vi "Code Page Table.vi"() -> (3 "Code Page Table":T1(array[cluster])=[{"Name"="Thai", "Tag"="th", "Code Page"=874}, {"Name"="Japanese", "Tag"="ja", "Code Page"=932}, {"Name"="Chinese (Simp)", "Tag"="zh-cn", "Code Page"=936}, {"Name"="Korean", "Tag"="ko", "Code Page"=949}, {"Name"="Chinese (Trad)", "Tag"="zh-tw", "Code Page"=950}, {"Name"="Czech", "Tag"="cs", "Code Page"=1250}, {"Name"="Slovak", "Tag"="sk", "Code Page"=1250}, {"Name"="Polish", "Tag"="pl", "Code Page"=1250}, {"Name"="Hungarian", "Tag"="hu", "Code Page"=1250}, {"Name"="Slovene", "Tag"="sl", "Code Page"=1250}, {"Name"="Bosnian", "Tag"="bs", "Code Page"=1250}, {"Name"="Croatian", "Tag"="hr", "Code Page"=1250}, {"Name"="Serbian", "Tag"="sr", "Code Page"=1250}, {"Name"="Romanian", "Tag"="ro", "Code Page"=1250}, {"Name"="Albanian", "Tag"="sq", "Code Page"=1250}, {"Name"="Russian", "Tag"="ru", "Code Page"=1251}, {"Name"="Bulgarian", "Tag"="bg", "Code Page"=1251}, {"Name"="Macedonian", "Tag"="mk", "Code Page"=1251}, {"Name"="Ukrainian", "Tag"="uk", "Code Page"=1251}, {"Name"="Afrikaans", "Tag"="af", "Code Page"=1252}, {"Name"="Basque", "Tag"="eu", "Code Page"=1252}, {"Name"="Catalan", "Tag"="ca", "Code Page"=1252}, {"Name"="Danish", "Tag"="da", "Code Page"=1252}, {"Name"="Dutch", "Tag"="nl", "Code Page"=1252}, {"Name"="English", "Tag"="en", "Code Page"=1252}, {"Name"="Faroese", "Tag"="fo", "Code Page"=1252}, {"Name"="Finnish", "Tag"="fi", "Code Page"=1252}, {"Name"="French", "Tag"="fr", "Code Page"=1252}, {"Name"="Galician", "Tag"="gl", "Code Page"=1252}, {"Name"="German", "Tag"="ge", "Code Page"=1252}, {"Name"="Icelandic", "Tag"="is", "Code Page"=1252}, {"Name"="Irish", "Tag"="ga", "Code Page"=1252}, {"Name"="Italian", "Tag"="it", "Code Page"=1252}, {"Name"="Norwegian", "Tag"="no", "Code Page"=1252}, {"Name"="Portuguese", "Tag"="pt", "Code Page"=1252}, {"Name"="Scottish", "Tag"="gd", "Code Page"=1252}, {"Name"="Spanish", "Tag"="es", "Code Page"=1252}, {"Name"="Swedish", "Tag"="sv", "Code Page"=1252}, {"Name"="Greek", "Tag"="el", "Code Page"=1253}, {"Name"="Turkish", "Tag"="tr", "Code Page"=1254}, {"Name"="Hebrew", "Tag"="he", "Code Page"=1255}, {"Name"="Farsi", "Tag"="fa", "Code Page"=1256}, {"Name"="Latvian", "Tag"="lv", "Code Page"=1257}, {"Name"="Lithuanian", "Tag"="lt", "Code Page"=1257}, {"Name"="Estonian", "Tag"="et", "Code Page"=1257}, {"Name"="Vietnamese", "Tag"="vt", "Code Page"=1258}])   [LabVIEW 2013, in "SET Project Data.lvlib"]
uses:
  SET Project Data.lvlib
panel:
  # "List of all supported languages. This should be stored in a config file but this should\ndo for now."
  # "Sources:\n1) List of ISO 639-1 codes - Wikipedia, the free encyclopedia\nhttp://en.wikipedia.org/wiki/List_of_ISO_639-1_codes\n\n2) Israel Science and Technology Homepage - Windows Locale Codes - Sortable list\nhttp://www.science.co.il/Language/Locale-codes.asp"
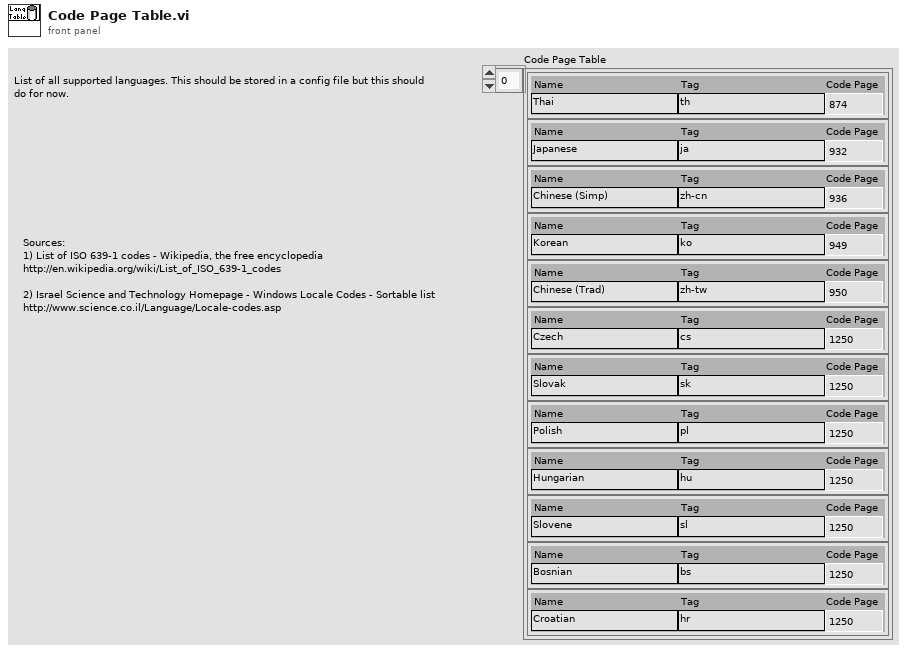
[diagram p1: front panel]
types:
  T1 = cluster{"Name":string, "Tag":string, "Code Page":u16}[]
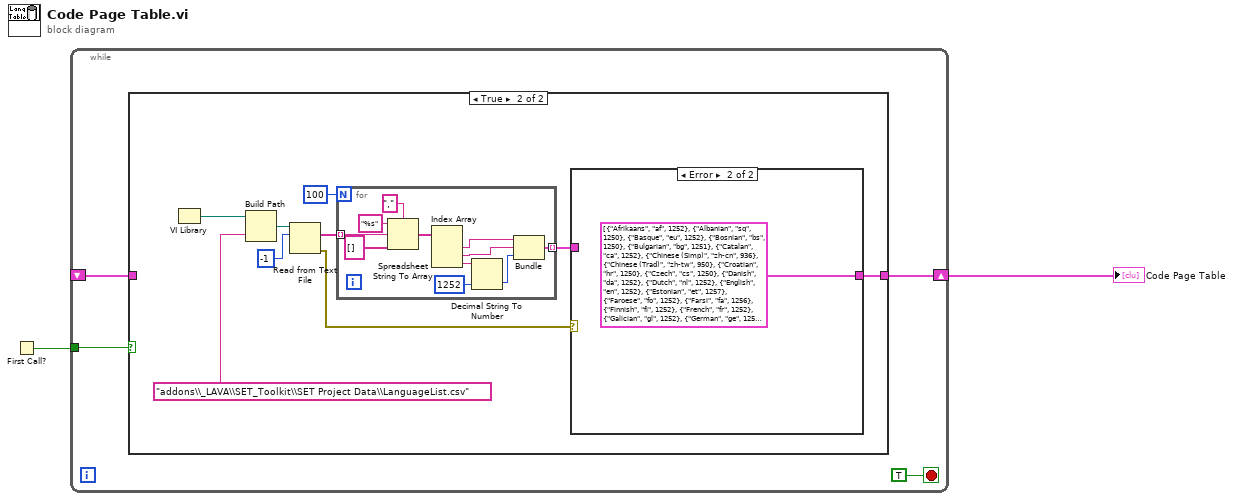
[diagram p0: block diagram]
diagram:
  n1 = First Call?() -> (First Call?: T/F=w1:bool)
  n2 = while {
    tunnel: w1 -> [w5]
    shift-right: [w6] -> w2
    shift-left: _ -> [w3]
    stop <- TRUE stop-if-true
    n3 = case shown="True" w5 {
      tunnel: [w7 w16] -> w6
      tunnel: w3 -> [w7 _]
      frame False {
      }
      frame True {
        n4 = VI Library() -> (path=w9:path)
        n5 = Build Path(base path=w9, name or relative path="addons\\_LAVA\\SET_Toolkit\\SET Project Data\\LanguageList.csv") -> (appended path=w15:path)
        n6 = Read from Text File(file (use dialog)=w15, count=-1) -> (text=w13:string[], error out=w11:errorcluster)  [unwired: 2 in, 2 out]
        n7 = for {
          N: 100 -> [_]
          tunnel: w13 -> [w27] mode=indexing
          tunnel: [w18] -> w12 mode=indexing
          n8 = Spreadsheet String To Array(delimiter (Tab)=",", format string="%s" ("format (%.3f)"), spreadsheet string=w27, array type (2D Dbl)=string[] []) -> (array=w24:string[])
          n9 = Index Array(array=w24) -> (element #1=w21:string, element #2=w20:string, element #3=w23:string)  [unwired: 3 in]
          n10 = Decimal String To Number(string=w23, default (0L)=1252 ("Code Page")) -> (number=w19:i32)  [unwired: 1 in, 1 out]
          n11 = Bundle(w21, w20, w19) -> (w18:cluster{string, string, i32})  [unwired: 1 in]
        }
        n12 = case shown="Error" w11 {
          tunnel: [w28 T1 [{"Name"="Afrikaans", "Tag"="af", "Code Page"=1252}, {"Name"="Albanian", "Tag"="sq", "Code Page"=1250}, {"Name"="Basque", "Tag"="eu", "Code Page"=1252}, {"Name"="Bosnian", "Tag"="bs", "Code Page"=1250}, {"Name"="Bulgarian", "Tag"="bg", "Code Page"=1251}, {"Name"="Catalan", "Tag"="ca", "Code Page"=1252}, {"Name"="Chinese (Simp)", "Tag"="zh-cn", "Code Page"=936}, {"Name"="Chinese (Trad)", "Tag"="zh-tw", "Code Page"=950}, {"Name"="Croatian", "Tag"="hr", "Code Page"=1250}, {"Name"="Czech", "Tag"="cs", "Code Page"=1250}, {"Name"="Danish", "Tag"="da", "Code Page"=1252}, {"Name"="Dutch", "Tag"="nl", "Code Page"=1252}, {"Name"="English", "Tag"="en", "Code Page"=1252}, {"Name"="Estonian", "Tag"="et", "Code Page"=1257}, {"Name"="Faroese", "Tag"="fo", "Code Page"=1252}, {"Name"="Farsi", "Tag"="fa", "Code Page"=1256}, {"Name"="Finnish", "Tag"="fi", "Code Page"=1252}, {"Name"="French", "Tag"="fr", "Code Page"=1252}, {"Name"="Galician", "Tag"="gl", "Code Page"=1252}, {"Name"="German", "Tag"="ge", "Code Page"=1252}, {"Name"="Greek", "Tag"="el", "Code Page"=1253}, {"Name"="Hebrew", "Tag"="he", "Code Page"=1255}, {"Name"="Hungarian", "Tag"="hu", "Code Page"=1250}, {"Name"="Icelandic", "Tag"="is", "Code Page"=1252}, {"Name"="Irish", "Tag"="ga", "Code Page"=1252}, {"Name"="Italian", "Tag"="it", "Code Page"=1252}, {"Name"="Japanese", "Tag"="ja", "Code Page"=932}, {"Name"="Korean", "Tag"="ko", "Code Page"=949}, {"Name"="Latvian", "Tag"="lv", "Code Page"=1257}, {"Name"="Lithuanian", "Tag"="lt", "Code Page"=1257}, {"Name"="Macedonian", "Tag"="mk", "Code Page"=1251}, {"Name"="Norwegian", "Tag"="no", "Code Page"=1252}, {"Name"="Polish", "Tag"="pl", "Code Page"=1250}, {"Name"="Portuguese", "Tag"="pt", "Code Page"=1252}, {"Name"="Romanian", "Tag"="ro", "Code Page"=1250}, {"Name"="Russian", "Tag"="ru", "Code Page"=1251}, {"Name"="Scottish", "Tag"="gd", "Code Page"=1252}, {"Name"="Serbian", "Tag"="sr", "Code Page"=1250}, {"Name"="Slovak", "Tag"="sk", "Code Page"=1250}, {"Name"="Slovene", "Tag"="sl", "Code Page"=1250}, {"Name"="Spanish", "Tag"="es", "Code Page"=1252}, {"Name"="Swedish", "Tag"="sv", "Code Page"=1252}, {"Name"="Thai", "Tag"="th", "Code Page"=874}, {"Name"="Turkish", "Tag"="tr", "Code Page"=1254}, {"Name"="Ukrainian", "Tag"="uk", "Code Page"=1251}, {"Name"="Vietnamese", "Tag"="vi", "Code Page"=1258}] ("Code Page Table")] -> w16
          tunnel: w12 -> [w28 _]
          frame No Error {
          }
          frame Error {
          }
        }
      }
    }
  }
  "Code Page Table" <- w2
